vi "GetValue.vi"(0 "VI Reference":refnum<vi>, 7 "Control Name":string, 11 "error in":errorcluster) -> (4 "VI Reference out":refnum<vi>, 8 "Control Value":variant, 15 "error out":errorcluster)   [LabVIEW 2016]
doc: "This VI gets the value of top level controls in other VI"
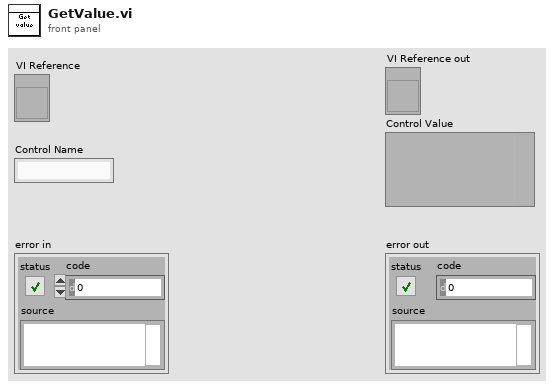
[diagram p1: front panel]
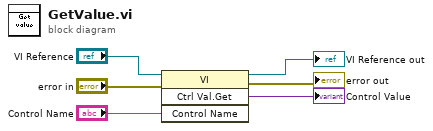
[diagram p0: block diagram]
diagram:
  n1 = invoke class="VI" method="Ctrl Val.Get"(reference="VI Reference", error in="error in", "Control Name"="Control Name") -> (reference out=→"VI Reference out":refnum<vi>, error out=→"error out":errorcluster, "Get Control Value Variant"=→"Control Value":variant)  [unwired: 1 in, 1 out]
